vi "PM5000_DateTime.vi"(8 "error in":errorcluster, 11 "Network Path":string="172.22.26.202") -> (0 "error out":errorcluster, 1 "TIEMPO_MEDICION":string, 2 "DateTime":T1, 3 "Network Path out":string="192.168.169.1")   [LabVIEW 2018]
doc: "Lee la tabla de memoria RealTime_VIF_Power del equipo PowerMonitor 5000, ademas filtra y ordena las variables de interez de la tabla de memoria.\n\nLee las siguientes variables de la tabla RealTime_VIF_Power:\n\n*V1_V2_Volts\n*V2_V3_Volts\n*V3_V1_Volts\n*I1_Amps\n*I2_Amps\n*I3_Amps\n*Frequency_Hz\n*Total_kW\n*Total_kVAR\n*Total_kVA\n*Total_True_PF\n*Total_Disp_PF"
uses:
  Controls/Date Time cluster.ctl
  <vilib>/ethernetip/ethernetip.llb/EthernetIP SLC500 Read Integer.vi
  <vilib>/ethernetip/ethernetip.lvlib
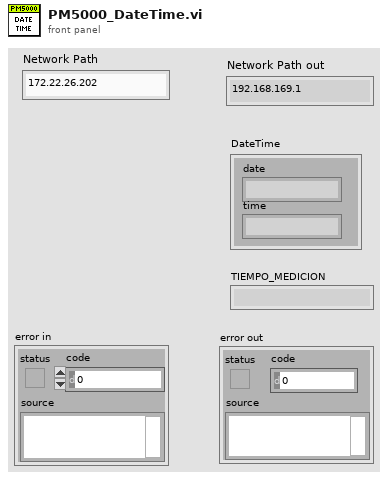
[diagram p1: front panel]
types:
  T1 = typedef "Date Time cluster.ctl" = cluster{"date":string, "time":string}
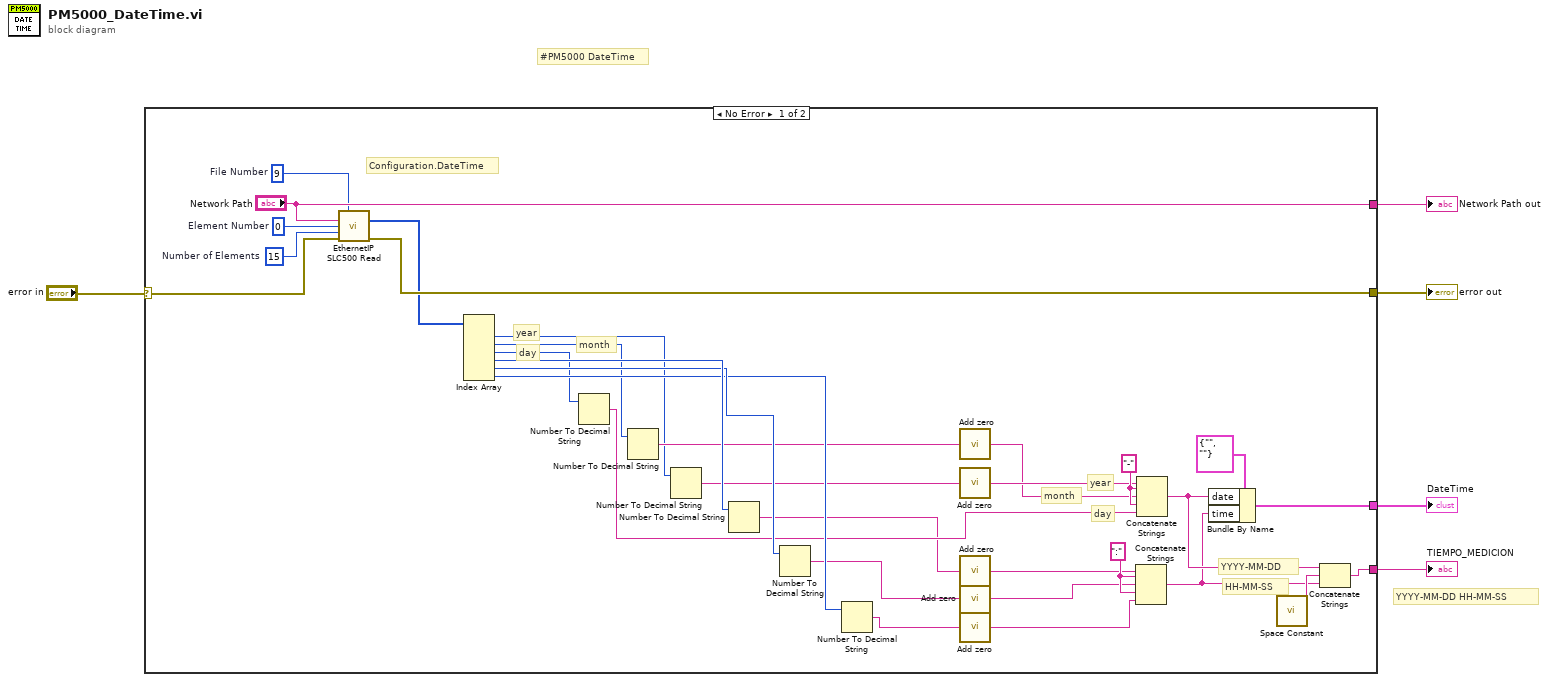
[diagram p0: block diagram]
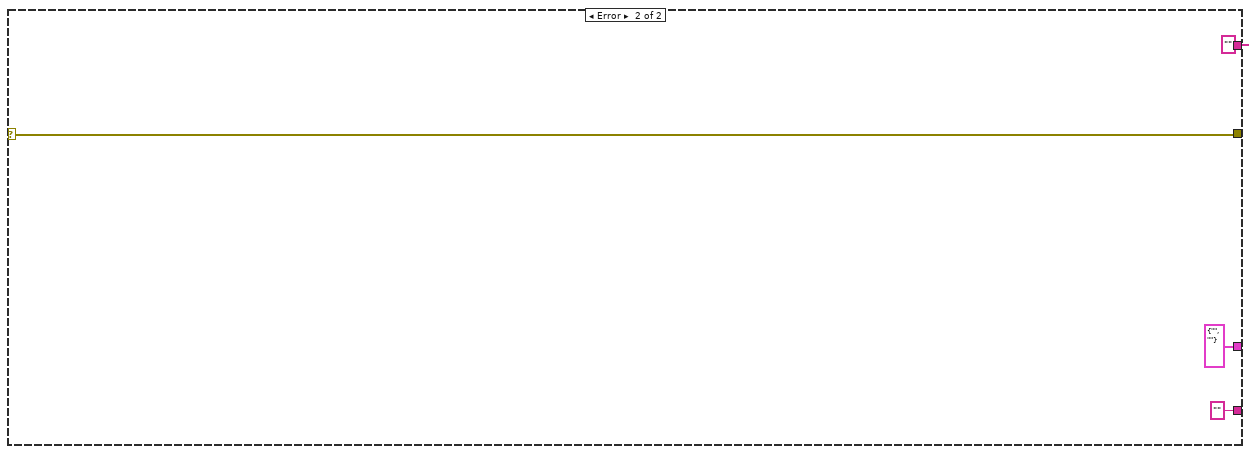
[diagram p2: hidden frame]
diagram:
  # "YYYY-MM-DD HH-MM-SS"
  # "#PM5000 DateTime"
  n1 = case shown="No Error" "error in" {
    selector: "error in" -> [w32 w40]
    tunnel: [w37 w40] -> w5
    tunnel: ["Network Path" "" ("Network Path")] -> w4
    tunnel: [w13 T1 {"date"="", "time"=""} ("DateTime")] -> w2
    tunnel: [w9 ""] -> w1
    frame No Error {
      w29 = ":"
      w30 = "-"
      w33 = u32 15  # Number of Elements
      w35 = u16 9  # File Number
      w34 = u16 0  # Element Number
      # "HH-MM-SS"
      # "day"
      # "month"
      # "year"
      # "YYYY-MM-DD"
      # "year"
      # "month"
      # "day"
      # "Configuration.DateTime"
      n2 = call-poly <vilib>:"EthernetIP SLC500 Read.vi"("File Number"=w35, "Network Path"="Network Path", "Element Number"=w34, "Number of Elements"=w33, "error in"=w32) -> ("Data"=w31:i16[], "error out"=w37:errorcluster)  [unwired: 8 in, 1 out]
      n3 = Index Array(array=w31) -> (element #1=w8:i16, element #2=w7:i16, element #3=w6:i16, element #4=w28:i16, element #5=w27:i16, element #6=w26:i16)  [unwired: 6 in]
      n4 = Number To Decimal String(number=w6) -> (decimal integer string=w24:string)  [unwired: 1 in]
      n5 = Number To Decimal String(number=w7) -> (decimal integer string=w25:string)  [unwired: 1 in]
      n6 = Number To Decimal String(number=w8) -> (decimal integer string=w23:string)  [unwired: 1 in]
      n7 = Number To Decimal String(number=w28) -> (decimal integer string=w20:string)  [unwired: 1 in]
      n8 = Number To Decimal String(number=w27) -> (decimal integer string=w18:string)  [unwired: 1 in]
      n9 = Number To Decimal String(number=w26) -> (decimal integer string=w16:string)  [unwired: 1 in]
      n10 = call "Add zero.vi"("in"=w25) -> ("out"=w21:string)
      n11 = call "Add zero.vi"("in"=w23) -> ("out"=w22:string)
      n12 = call "Add zero.vi"("in"=w20) -> ("out"=w19:string)
      n13 = call "Add zero.vi"("in"=w18) -> ("out"=w17:string)
      n14 = call "Add zero.vi"("in"=w16) -> ("out"=w15:string)
      n15 = Concatenate Strings(w19, w29, w17, w29, w15) -> (w10:string)
      n16 = Concatenate Strings(w22, w30, w21, w30, w24) -> (w11:string)
      n17 = Bundle By Name(cluster=T1 {"date"="", "time"=""} ("DateTime"), "date"=w11, "time"=w10) -> (w13:T1)
      n18 = call <vilib>:"Space Constant.vi"() -> ("String"=w12:string)
      n19 = Concatenate Strings(w11, w12, w10) -> (w9:string)
    }
    frame Error {
    }
  }
  "error out" <- w5
  "Network Path out" <- w4
  "DateTime" <- w2
  "TIEMPO_MEDICION" <- w1
